vi "checkForceErrorInRange.vi"(8 "error in (no error)":errorcluster, 11 "SystemController in":refnum<class "SystemController.lvclass">) -> (0 "error out":errorcluster, 2 "forceErrorInRangeIsTrue":bool, 3 "SystemController out":refnum<class "SystemController.lvclass">)   [LabVIEW 2013, in "SystemController.lvclass"]
uses:
  SystemController.lvclass
  SystemController.lvclass/SystemController.ctl
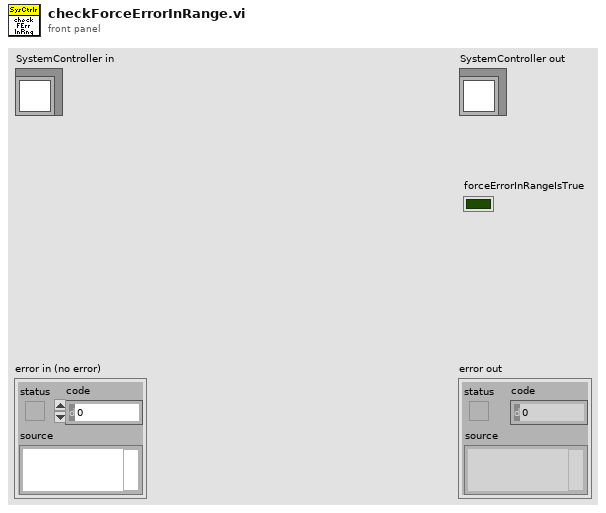
[diagram p1: front panel]
types:
  T1 = typedef "M2AADTTypedefs.lvlib/ForceDemand.ctl" = dbl[unit]
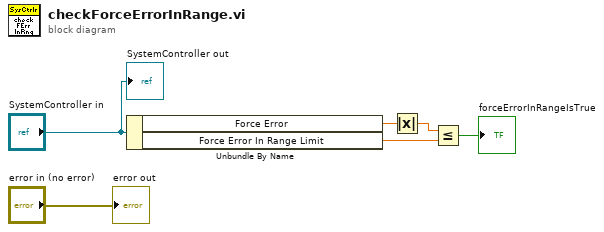
[diagram p0: block diagram]
diagram:
  n1 = Unbundle By Name("SystemController in") -> ("Force Error"=w4:T1, "Force Error In Range Limit"=w3:dbl[unit])
  n2 = Absolute Value(x=w4) -> (abs(x)=w2:T1)
  n3 = Less Or Equal?(x=w2, y=w3) -> (x <= y?=→"forceErrorInRangeIsTrue":bool)
  "error out" <- "error in (no error)"
  "SystemController out" <- "SystemController in"
